vi "EMG_DESC_main_v001.vi"() -> ()   [LabVIEW 2019]
uses:
  <vilib>/Utility/file.llb/Read Delimited Spreadsheet (DBL).vi
  <vilib>/Utility/file.llb/Read Delimited Spreadsheet (string).vi
panel:
  out "Impoting Path":path
  out "Waveform Graph":waveform(dbl)[](graph)
  in  "Samping Frequency":dbl=2000.0
  out "Headers":string[](array[string])
  out "Data":dbl[][](array[numeric])
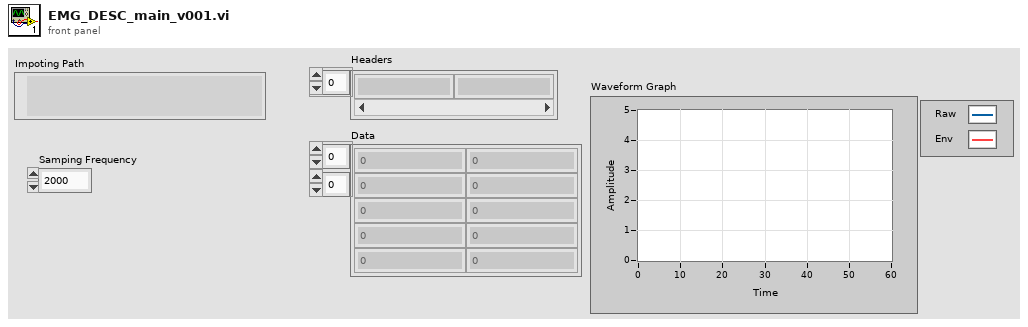
[diagram p1: front panel]
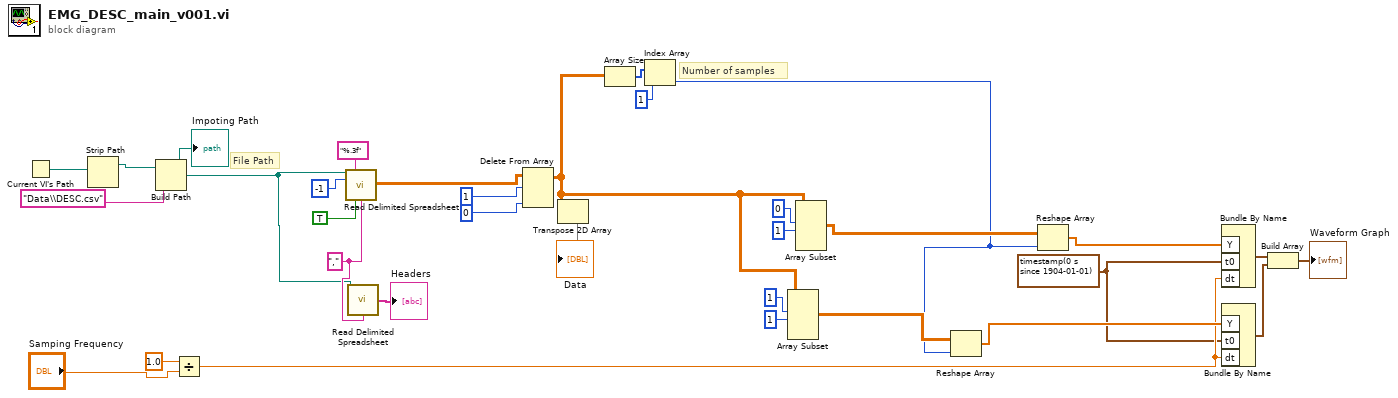
[diagram p0: block diagram]
diagram:
  w1 = timestamp(0 s since 1904-01-01) ("t0")
  w29 = "," ("delimiter (\\t)")
  # "File Path"
  # "Number of samples"
  n1 = Current VI's Path() -> (path=w8:path)
  n2 = Strip Path(path=w8) -> (stripped path=w7:path)  [unwired: 1 out]
  n3 = Build Path(base path=w7, name or relative path="Data\\DESC.csv") -> (appended path=w6:path)
  "Impoting Path" <- w6
  n4 = Divide(x=1.0, y="Samping Frequency") -> (x/y=w5:dbl)
  n5 = call-poly <vilib>:"Read Delimited Spreadsheet.vi"("file path (dialog if empty)"=w6, "format (%.3f)"="%.3f", "number of rows (all:-1)"=-1, "transpose? (F)"=TRUE, "delimiter (\\t)"=w29) -> ("all rows"=w25:dbl[][])  [unwired: 5 in, 5 out]
  n6 = call-poly <vilib>:"Read Delimited Spreadsheet.vi"("file path (dialog if empty)"=w6, "delimiter (\\t)"=w29) -> ("first row"=→"Headers":string[])  [unwired: 8 in, 5 out]
  n7 = Delete From Array(array=w25, length=1 ("index"), index (col)=0 ("index")) -> (array with subset deleted=w3:dbl[][])  [unwired: 1 in, 1 out]
  n8 = Transpose 2D Array(2D array=w3) -> (transposed array=→"Data":dbl[][])
  n9 = Array Size(array=w3) -> (size(s)=w22:i32[])
  n10 = Index Array(array=w22, index=1) -> (element=w2:i32)
  n11 = Array Subset(array=w3, index (row)=1 ("index"), length (row)=1 ("length")) -> (w13:dbl[][])  [unwired: 2 in]
  n12 = Array Subset(array=w3, index (row)=0 ("index"), length (row)=1 ("length")) -> (w16:dbl[][])  [unwired: 2 in]
  n13 = Reshape Array(w13, w2) -> (w14:dbl[])
  n14 = Reshape Array(w16, w2) -> (w15:dbl[])
  n15 = Bundle By Name("Y"=w15, "t0"=w1, "dt"=w5) -> (w12:waveform(dbl))  [unwired: 1 in]
  n16 = Bundle By Name("Y"=w14, "t0"=w1, "dt"=w5) -> (w11:waveform(dbl))  [unwired: 1 in]
  n17 = Build Array(w12, w11) -> (→"Waveform Graph":waveform(dbl)[])
